vi "Create.vi"(11 "Dev Actor Panel in":refnum<class "Dev Panel.lvclass">) -> (0 "error out":errorcluster, 3 "Dev Actor Panel out":refnum<class "Dev Panel.lvclass">)   [LabVIEW 2021, in "Dev Panel.lvclass"]
uses:
  Dev Panel.lvclass
  Dev Panel.lvclass/Dev Panel.ctl
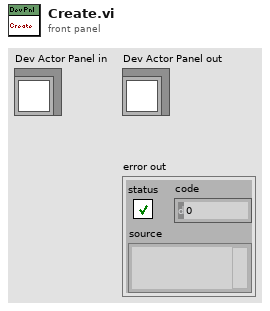
[diagram p1: front panel]
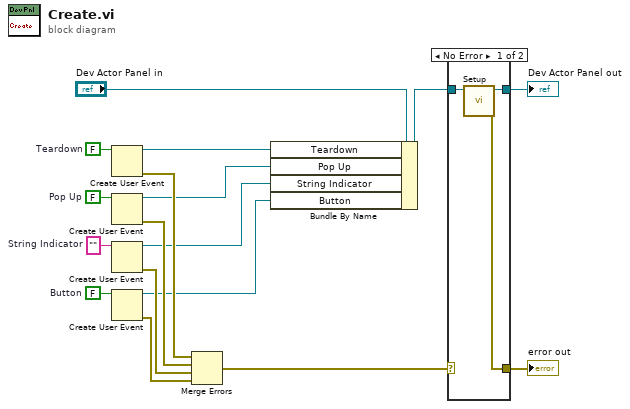
[diagram p0: block diagram]
diagram:
  w11 = FALSE  # Pop Up
  w12 = FALSE  # Button
  w13 = ""  # String Indicator
  w16 = FALSE  # Teardown
  n1 = Create User Event(user event datatype=w16) -> (user event=w15:refnum<user-event>, error out=w14:errorcluster)  [unwired: 1 in]
  n2 = Create User Event(user event datatype=w11) -> (user event=w7:refnum<user-event>, error out=w10:errorcluster)  [unwired: 1 in]
  n3 = Create User Event(user event datatype=w13) -> (user event=w6:refnum<user-event>, error out=w8:errorcluster)  [unwired: 1 in]
  n4 = Create User Event(user event datatype=w12) -> (user event=w5:refnum<user-event>, error out=w9:errorcluster)  [unwired: 1 in]
  n5 = Merge Errors(w14, w10, w8, w9) -> (w2:errorcluster)
  n6 = Bundle By Name(cluster="Dev Actor Panel in", "Teardown"=w15, "Pop Up"=w7, "String Indicator"=w6, "Button"=w5) -> (w4:refnum<class "Dev Panel.lvclass">)
  n7 = case shown="No Error" w2 {
    selector: w2 -> [_ w22]
    tunnel: w4 -> [w20 w21]
    tunnel: [w19 w21] -> w3
    tunnel: [w18 w22] -> w1
    frame No Error {
      n8 = call "Setup.vi"("Dev Panel in"=w20) -> ("error out"=w18:errorcluster, "Dev Panel out"=w19:refnum<class "Dev Panel.lvclass">)  [unwired: 9 in]
    }
    frame Error {
    }
  }
  "error out" <- w1
  "Dev Actor Panel out" <- w3
